vi "Picomotor UI.vi"() -> ()   [LabVIEW 2019]
uses:
  C:/Users/tungc/Desktop/OLED_Lab/controller/Samples/CmdLib.dll
  CmdLib.dll
  Global Variables.vi
panel:
  out "size(s)":i32
  in  "pos":i32
  out "CmdLib Out":refnum<k24>
  in  "CmdLib In":refnum<k24>
  in  "Selected Motor:":string(combo)
  out "CmdLib":refnum<k24>
  out "Status:":string
  in  "Relative Move 2-4:":string
  in  "Relative Move 2-3:":string
  in  "Relative Move 2-2:":string
  in  "Relative Move 2-1:":string
  in  "Relative Move 1-4:":string
  in  "Relative Move 1-3:":string
  in  "Relative Move 1-2:":string
  in  "Relative Move 1-1:":string
  out "Position status 2-3:":string
  out "Position status 2-2:":string
  out "Position status 2-4:":string
  out "Position status 2-1:":string
  in  "Selected Controller 2:":string(combo)
  in  "Selected Controller 1:":string(combo)
  out "Device Address":dbl
  out "Device Key":string[](array[string])
  out "Position status 1-3:":string
  out "Position status 1-2:":string
  out "Position status 1-4:":string
  out "Position status 1-1:":string
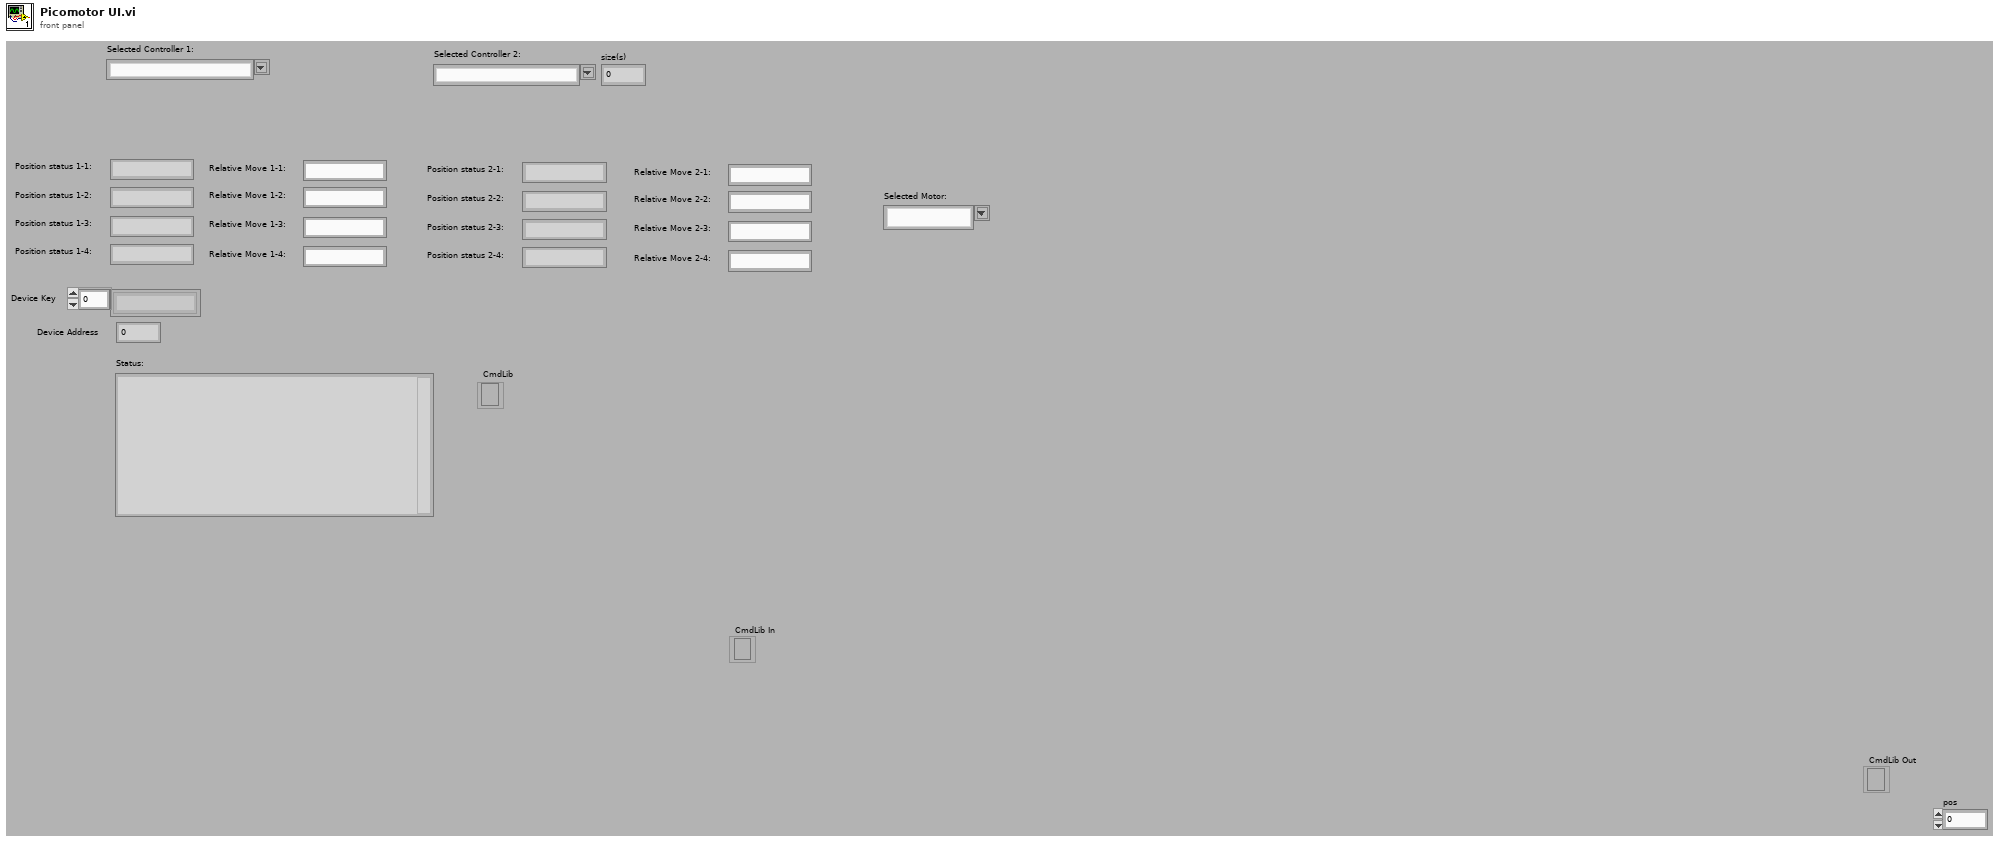
[diagram p1: front panel]
types:
  T1 = cluster{"Device Key":string, "GetMasterDeviceAddress":i32, string}
  T2 = cluster{"Device Key":string, "GetMasterDeviceAddress":i32, string}[]
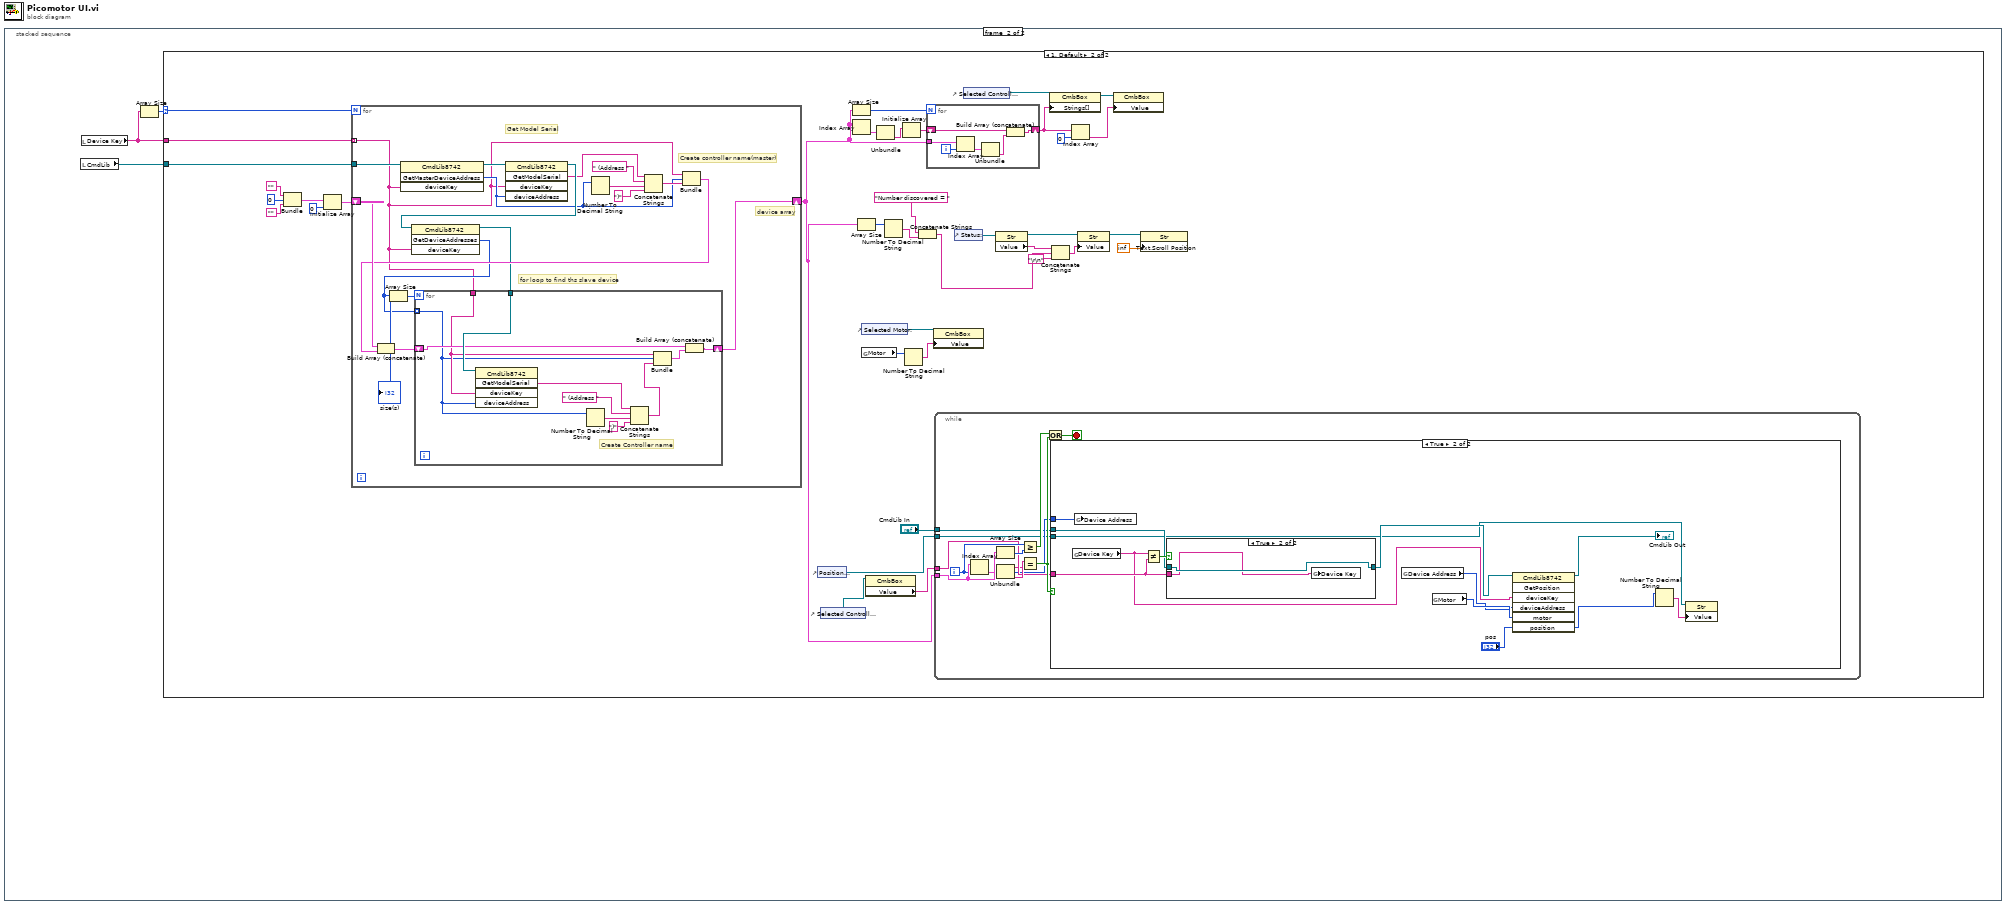
[diagram p0: block diagram]
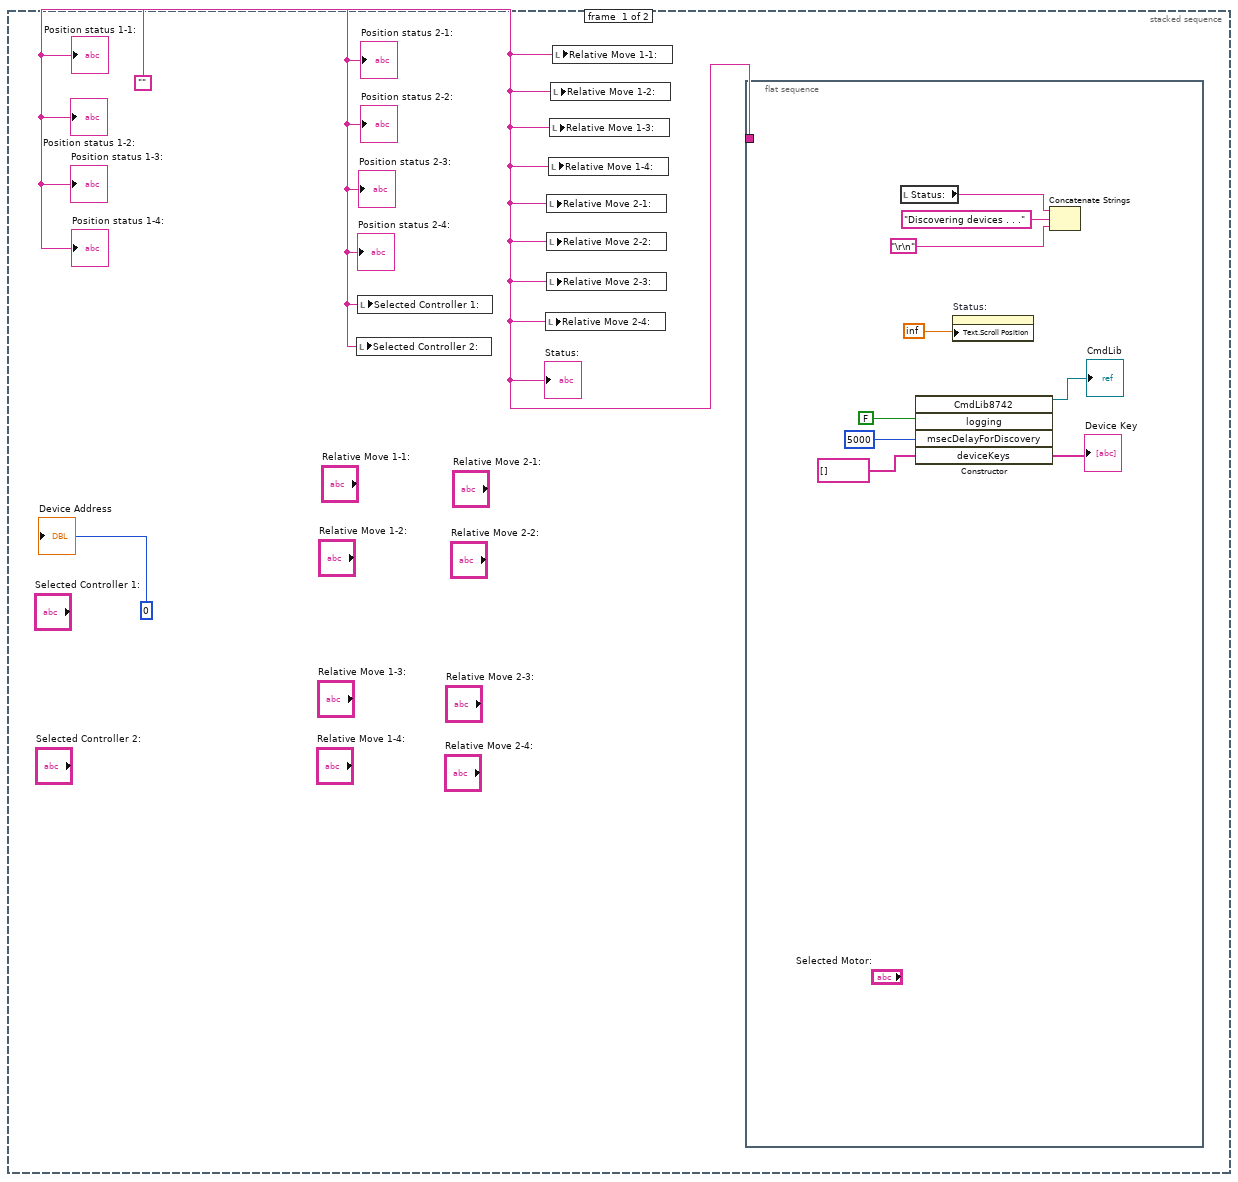
[diagram p2: hidden frame]
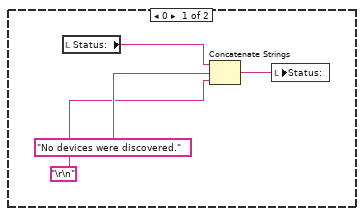
[diagram p3: hidden frame]
diagram:
  n1 = stacked-sequence {
    frame #0 {
      w1 = ""
      n2 = local write "Selected Controller 2:"(w1) -> ()
      n3 = local write "Selected Controller 1:"(w1) -> ()
      n4 = local write "Relative Move 2-4:"(w1) -> ()
      n5 = local write "Relative Move 2-1:"(w1) -> ()
      n6 = local write "Relative Move 2-2:"(w1) -> ()
      n7 = local write "Relative Move 2-3:"(w1) -> ()
      n8 = local write "Relative Move 1-4:"(w1) -> ()
      n9 = local write "Relative Move 1-3:"(w1) -> ()
      n10 = local write "Relative Move 1-2:"(w1) -> ()
      n11 = local write "Relative Move 1-1:"(w1) -> ()
      n12 = flat-sequence {
        tunnel: w1 -> [_]
        frame #0 {
          n13 = local read "Status:"() -> (w10:string)
          n14 = constructor class="CmdLib8742"("logging"=FALSE, "msecDelayForDiscovery"=5000, "deviceKeys"=string[] [] ("current density list")) -> (reference out=→"CmdLib":refnum<k24>, "deviceKeys"=→"Device Key":string[])  [unwired: 3 in, 4 out]
          n15 = property on="Status:" class="Str"("Text.Scroll Position"=inf) -> ()  [unwired: 2 in, 2 out]
          n16 = Concatenate Strings(w10, "Discovering devices . . ." ("Input String"), "\r\n") -> ()  [unwired: 1 out]
        }
      }
      "Position status 1-1:" <- w1
      "Position status 1-4:" <- w1
      "Position status 1-2:" <- w1
      "Position status 1-3:" <- w1
      "Device Address" <- 0
      "Position status 2-1:" <- w1
      "Position status 2-4:" <- w1
      "Position status 2-2:" <- w1
      "Position status 2-3:" <- w1
      "Status:" <- w1
    }
    frame #1 {
      n17 = local read "CmdLib"() -> (w13:refnum<k24>)
      n18 = local read "Device Key"() -> (w14:string[])
      n19 = Array Size(array=w14) -> (size(s)=w12:i32)
      n20 = case shown="1, Default" w12 {
        selector: w12 -> [_ w50]
        tunnel: w14 -> [_ w47]
        tunnel: w13 -> [_ w48]
        frame 0 {
          n21 = local read "Status:"() -> (w16:string)
          n22 = Concatenate Strings(w16, "No devices were discovered." ("Input String"), "\r\n") -> (w15:string)
          n23 = local write "Status:"(w15) -> ()
        }
        frame 1, Default {
          n24 = Bundle("", 0, "") -> (w52:cluster{string, i32, string})  [unwired: 1 in]
          n25 = Initialize Array(w52, 0 ("dimension size")) -> (w49:cluster{string, i32, string}[])
          n26 = for {
            N: w50 -> [_]
            shift-right: [w91] -> w21
            shift-left: w49 -> [w98]
            tunnel: w48 -> [w107]
            tunnel: w47 -> [w92] mode=indexing
            # "device array"
            # "for loop to find ths slave device"
            # "Create controller name(master)"
            # "Get Model Serial"
            n27 = invoke class="CmdLib8742" method="GetMasterDeviceAddress"(reference=w107, "deviceKey"=w92) -> (reference out=w106:refnum<k24>, "GetMasterDeviceAddress"=w99:i32)  [unwired: 2 in, 2 out]
            n28 = invoke class="CmdLib8742" method="GetModelSerial"(reference=w106, "deviceKey"=w92, "deviceAddress"=w99) -> (reference out=w105:refnum<k24>, "GetModelSerial"=w101:string)  [unwired: 2 in, 3 out]
            n29 = invoke class="CmdLib8742" method="GetDeviceAddresses"(reference=w105, "deviceKey"=w92) -> (reference out=w93:refnum<k24>, "GetDeviceAddresses"=w94:i32[])  [unwired: 2 in, 2 out]
            n30 = Array Size(array=w94) -> (size(s)=w95:i32)
            "size(s)" <- w95
            n31 = Number To Decimal String(number=w99) -> (decimal integer string=w104:string)  [unwired: 1 in]
            n32 = Concatenate Strings(w101, " (Address " ("string"), w104, ")" ("string")) -> (w100:string)
            n33 = Bundle("Device Key"=w92, "GetMasterDeviceAddress"=w99, w100) -> (w97:T1)  [unwired: 1 in]
            n34 = Build Array (concatenate)(w98, w97) -> (w96:T2)
            n35 = for {
              N: w95 -> [_]
              shift-right: [w113] -> w91
              shift-left: w96 -> [w112]
              tunnel: w94 -> [w109] mode=indexing
              tunnel: w93 -> [w118]
              tunnel: w92 -> [w110]
              # "Create Controller name"
              n36 = invoke class="CmdLib8742" method="GetModelSerial"(reference=w118, "deviceKey"=w110, "deviceAddress"=w109) -> ("GetModelSerial"=w114:string)  [unwired: 2 in, 4 out]
              n37 = Number To Decimal String(number=w109) -> (decimal integer string=w117:string)  [unwired: 1 in]
              n38 = Concatenate Strings(w114, " (Address " ("string"), w117, ")" ("string")) -> (w108:string)
              n39 = Bundle("Device Key"=w110, w109, w108) -> (w111:cluster{"Device Key":string, i32, string})  [unwired: 1 in]
              n40 = Build Array (concatenate)(w112, w111) -> (w113:T2)
            }
          }
          n41 = control-ref of="Position status 1-1:"() -> (w19:refnum<vi>)
          n42 = control-ref of="Selected Controller 1:"() -> (w20:refnum<vi>)
          n43 = Array Size(array=w21) -> (size(s)=w43:i32)
          n44 = Index Array(array=w21) -> (element=w42:cluster{string, i32, string})  [unwired: 1 in]
          n45 = Array Size(array=w21) -> (size(s)=w38:i32)
          n46 = control-ref of="Selected Motor:"() -> (w24:refnum<vi>)
          n47 = global read "Global Variables.vi" "Motor"() -> (w25:i32)
          n48 = property class="CmbBox"(reference=w20) -> ("Value"=w23:string)  [unwired: 1 in, 2 out]
          n49 = Unbundle(w42) -> (w41:string)  [unwired: 2 out]
          n50 = Number To Decimal String(number=w38) -> (decimal integer string=w37:string)  [unwired: 1 in]
          n51 = Initialize Array(w41) -> (w40:string[])  [unwired: 1 in]
          n52 = Number To Decimal String(number=w25) -> (decimal integer string=w26:string)  [unwired: 1 in]
          n53 = Concatenate Strings("Number discovered = " ("string"), w37) -> (w29:string)
          n54 = for {
            N: w43 -> [_]
            tunnel: w21 -> [w90]
            shift-right: [w86] -> w39
            shift-left: w40 -> [w87]
            i -> [w89]
            n55 = Index Array(array=w90, index=w89) -> (element=w88:cluster{string, i32, string})
            n56 = Unbundle(w88) -> (w85:string)  [unwired: 2 out]
            n57 = Build Array (concatenate)(w87, w85) -> (w86:string[])
          }
          n58 = property class="CmbBox"(reference=w24, "Value"=w26) -> ()  [unwired: 1 in, 2 out]
          n59 = while {
            tunnel: w21 -> [w67]
            tunnel: w23 -> [w56]
            tunnel: w19 -> [w58]
            tunnel: "CmdLib In" -> [w57]
            i -> [w66]
            stop <- w61 stop-if-true
            n60 = Index Array(array=w67, index=w66) -> (element=w65:cluster{string, i32, string})
            n61 = Array Size(array=w67) -> (size(s)=w68:i32)
            n62 = Unbundle(w65) -> (w60:string, w59:i32, w64:string)
            n63 = Greater Or Equal?(x=w66, y=w68) -> (x >= y?=w63:bool)
            n64 = Equal?(x=w64, y=w56) -> (x = y?=w62:bool)
            n65 = Or(x=w63, y=w62) -> (x .or. y?=w61:bool)
            n66 = case shown="True" w62 {
              tunnel: w60 -> [_ w81]
              tunnel: w59 -> [_ w78]
              tunnel: w58 -> [_ w70]
              tunnel: w57 -> [_ w79]
              frame False {
              }
              frame True {
                n67 = global read "Global Variables.vi" "Device Key"() -> (w69:string)
                n68 = global write "Global Variables.vi" "Device Address"(w78) -> ()
                n69 = Not Equal?(x=w69, y=w81) -> (x != y?=w80:bool)
                n70 = case shown="True" w80 {
                  tunnel: w79 -> [w82 w84]
                  tunnel: w81 -> [_ w83]
                  tunnel: [w82 w84] -> w72
                  frame False {
                  }
                  frame True {
                    n71 = global write "Global Variables.vi" "Device Key"(w83) -> ()
                  }
                }
                n72 = global read "Global Variables.vi" "Device Address"() -> (w73:i32)
                n73 = global read "Global Variables.vi" "Motor"() -> (w74:i32)
                n74 = invoke class="CmdLib8742" method="GetPosition"(reference=w72, "deviceKey"=w69, "deviceAddress"=w73, "motor"=w74, "position"="pos") -> (reference out=→"CmdLib Out":refnum<k24>, "position"=w75:i32)  [unwired: 2 in, 5 out]
                n75 = Number To Decimal String(number=w75) -> (decimal integer string=w77:string)  [unwired: 1 in]
                n76 = property class="Str"(reference=w70, "Value"=w77) -> ()  [unwired: 1 in, 2 out]
              }
            }
          }
          n77 = control-ref of="Status:"() -> (w27:refnum<vi>)
          n78 = control-ref of="Selected Controller 1:"() -> (w28:refnum<vi>)
          n79 = property on="Property Node" class="Str"(reference=w27) -> (reference out=w32:refnum<vi>, "Value"=w34:string)  [unwired: 1 in, 1 out]
          n80 = property class="CmbBox"(reference=w28, "Strings[]"=w39) -> (reference out=w44:refnum<vi>)  [unwired: 1 in, 1 out]
          n81 = Concatenate Strings(w34, w29, "\r\n") -> (w33:string)
          n82 = Index Array(array=w39, index=0) -> (element=w46:string)
          n83 = property class="Str"(reference=w32, "Value"=w33) -> (reference out=w31:refnum<vi>)  [unwired: 1 in, 1 out]
          n84 = property class="CmbBox"(reference=w44, "Value"=w46) -> ()  [unwired: 1 in, 2 out]
          n85 = property class="Str"(reference=w31, "Text.Scroll Position"=inf) -> ()  [unwired: 1 in, 2 out]
        }
      }
    }
  }
